vi "ABR3-Estimate Threshold (wrapper).vi"(7 "Threshold Estimation":T4={"Tmin (ms)"=1.0, "Tmax (ms)"=6.0, "CC criterion"=0.35, "adjR2 criterion"=0.0}, 11 "error in (no error)":errorcluster, 12 "Analysis (in)":T3) -> (8 "Work":T1, 14 "Analysis (out)":T3, 15 "error out":errorcluster)   [LabVIEW 2020]
uses:
  TypeDefs/ABR3-Analysis State.ctl
  ABR3-Threshold Estimation Result.ctl
  ABR3-Threshold Estimation Parameters.ctl
  ABR3-Threshold Estimation Work.ctl
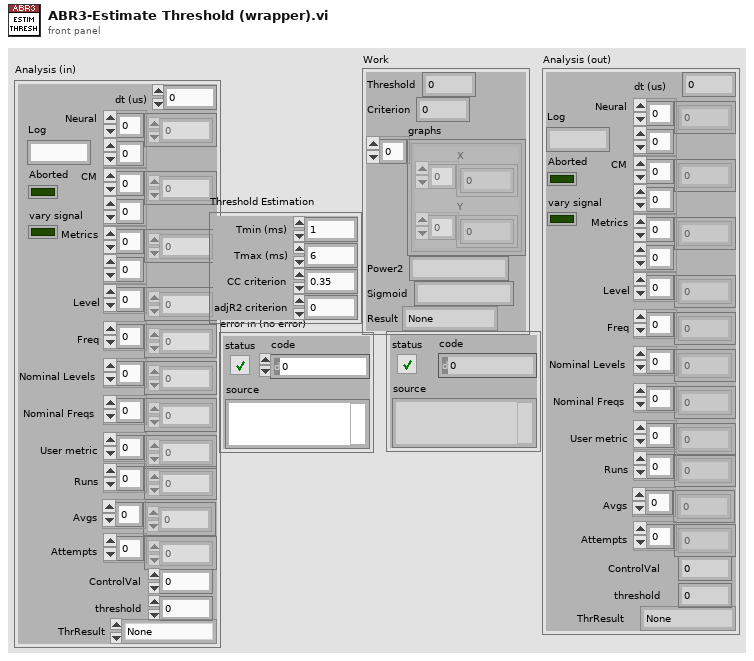
[diagram p1: front panel]
types:
  T1 = typedef "ABR3-Threshold Estimation Work.ctl" = cluster{"Threshold":dbl, "Criterion":dbl, "graphs":cluster{"X":dbl[], "Y":dbl[]}[], "Power2":string, "Sigmoid":string, "Result":T2}
  T2 = typedef "ABR3-Threshold Estimation Result.ctl" = enum16{"None", "Power", "Sigmoid", "Power (noisy)", "Suprathreshold", "Invalid"}
  T3 = typedef "ABR3-Analysis State.ctl" = cluster{"dt (us)":dbl, "Neural":dbl[][], "CM":dbl[][], "Metrics":dbl[][], "Level":dbl[], "Freq":dbl[], "Nominal Levels":dbl[], "Nominal Freqs":dbl[], "User metric":dbl[], "Runs":i32[], "Avgs":i32[], "Attempts":i32[], "Log":string, "Aborted":bool, "ControlVal":dbl, "threshold":dbl, "vary signal":bool, "ThrResult":T2}
  T4 = typedef "ABR3-Threshold Estimation Parameters.ctl" = cluster{"Tmin (ms)":dbl, "Tmax (ms)":dbl, "CC criterion":dbl, "adjR2 criterion":dbl}
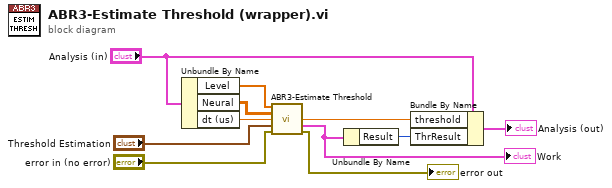
[diagram p0: block diagram]
diagram:
  n1 = Unbundle By Name("Analysis (in)") -> ("Level"=w9:dbl[], "Neural"=w8:dbl[][], "dt (us)"=w7:dbl)
  n2 = call "ABR3-Estimate Threshold.vi"("Level (in)"=w9, "Neural"=w8, "dt (us)"=w7, "Threshold Estimation"="Threshold Estimation", "error in (no error)"="error in (no error)") -> ("Threshold"=w4:dbl, "Work"=w2:T1, "error out"=→"error out":errorcluster)  [unwired: 8 in]
  "Work" <- w2
  n3 = Unbundle By Name(w2) -> ("Result"=w1:T2)
  n4 = Bundle By Name(cluster="Analysis (in)", "threshold"=w4, "ThrResult"=w1) -> (→"Analysis (out)":T3)
